vi "Close Instrument.vi"(8 "error in (no error)":errorcluster, 11 ".NET Refnum in":refnum<k24>) -> (0 "error out":errorcluster)   [LabVIEW 2019, in "ESP301.lvlib"]
uses:
  ESP301.lvlib
  Newport.ESP301.CommandInterface
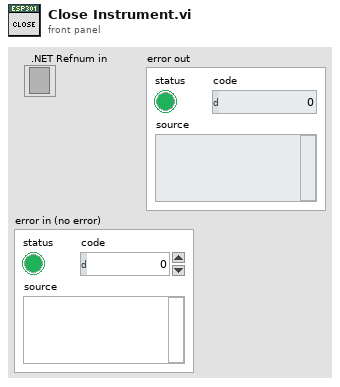
[diagram p1: front panel]
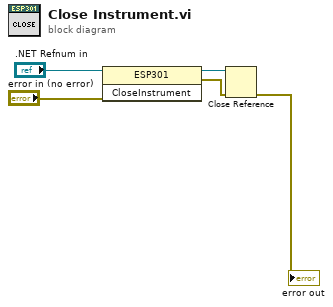
[diagram p0: block diagram]
diagram:
  n1 = invoke class="ESP301" method="CloseInstrument"(reference=".NET Refnum in", error in="error in (no error)") -> (reference out=w2:refnum<k24>, error out=w5:errorcluster)  [unwired: 1 in, 1 out]
  n2 = Close Reference(reference=w2, error in (no error)=w5) -> (error out=→"error out":errorcluster)
